vi "Find_Unsigned_Tracks-1.vi"(4 "error IN":errorcluster, 7 "Track ID IN":u16[](array[numeric])) -> (0 "error OUT":errorcluster, 2 "Position Mis ID":i32[](array[numeric]), 3 "Mistake ID":u16[](array[numeric]))   [LabVIEW 2013]
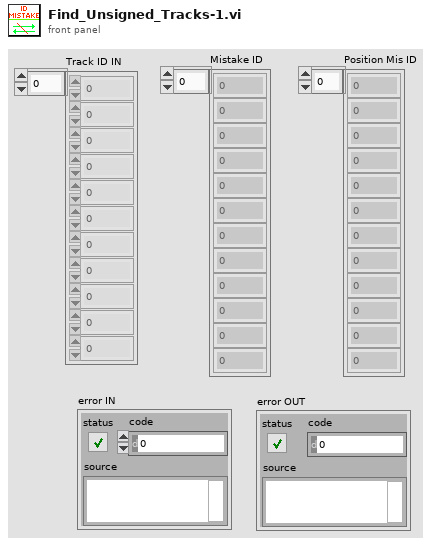
[diagram p1: front panel]
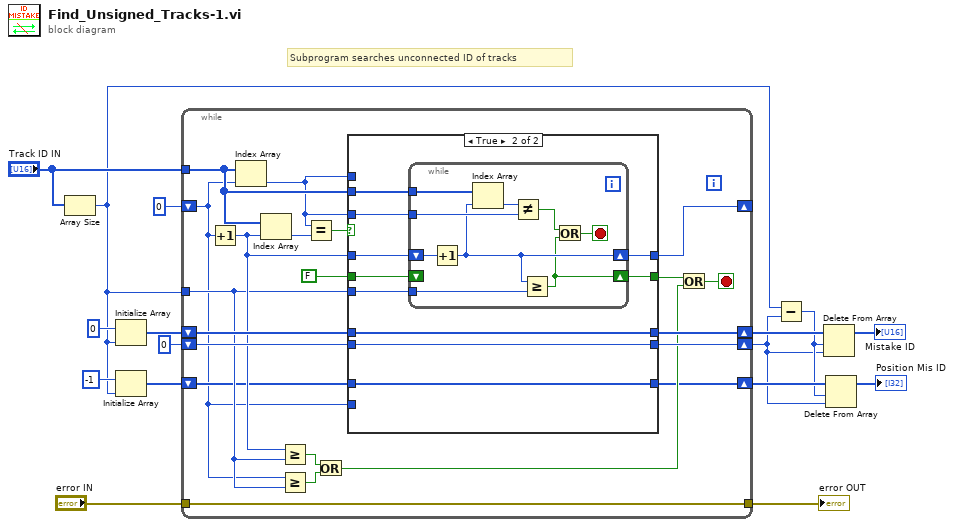
[diagram p0: block diagram]
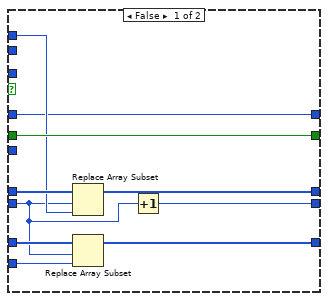
[diagram p2: hidden frame]
diagram:
  # "Subprogram searches unconnected ID of tracks"
  n1 = Array Size(array="Track ID IN") -> (size(s)=w6:i32)
  n2 = Initialize Array(u16 0 ("element"), w6) -> (w14:u16[])
  n3 = Initialize Array(-1 ("element"), w6) -> (w5:i32[])
  n4 = while {
    tunnel: "Track ID IN" -> [w35]
    shift-right: [w29] -> w10
    shift-left: w14 -> [w33]
    shift-right: [w23] -> _
    shift-left: 0 -> [w17]
    tunnel: w6 -> [w27]
    shift-right: [w30] -> w2
    shift-left: 0 -> [w32]
    tunnel: "error IN" -> [w24]
    tunnel: [w24] -> w9
    shift-right: [w18] -> w4
    shift-left: w5 -> [w19]
    stop <- w21 stop-if-true
    n5 = Increment(x=w17) -> (x+1=w28:i32)
    n6 = Index Array(array=w35, index=w17) -> (element=w31:u16)
    n7 = Index Array(array=w35, index=w28) -> (element=w37:u16)
    n8 = Greater Or Equal?(x=w28, y=w27) -> (x >= y?=w26:bool)
    n9 = Greater Or Equal?(x=w17, y=w27) -> (x >= y?=w25:bool)
    n10 = Equal?(x=w31, y=w37) -> (x = y?=w36:bool)
    n11 = Or(x=w26, y=w25) -> (x .or. y?=w20:bool)
    n12 = case shown="True" w36 {
      tunnel: w28 -> [w42 w57]
      tunnel: w35 -> [_ w56]
      tunnel: w31 -> [_ w55]
      tunnel: w27 -> [_ w54]
      tunnel: FALSE -> [w47 w53]
      tunnel: [w47 w50] -> w22
      tunnel: w33 -> [w46 w52]
      tunnel: w32 -> [w38 w51]
      tunnel: w31 -> [w45 _]
      tunnel: [w44 w51] -> w30
      tunnel: [w43 w52] -> w29
      tunnel: [w42 w49] -> w23
      tunnel: w19 -> [w41 w48]
      tunnel: [w40 w48] -> w18
      tunnel: w17 -> [w39 _]
      frame False {
        n13 = Replace Array Subset(array=w46, new element=w45, index=w38) -> (w43:u16[])
        n14 = Replace Array Subset(array=w41, new element=w39, index=w38) -> (w40:i32[])
        n15 = Increment(x=w38) -> (x+1=w44:i32)
      }
      frame True {
        n16 = while {
          shift-right: [w62] -> w49
          shift-left: w57 -> [w66]
          tunnel: w56 -> [w65]
          tunnel: w55 -> [w63]
          tunnel: w54 -> [w61]
          shift-right: [w58] -> w50
          shift-left: w53 -> [_]
          stop <- w59 stop-if-true
          n17 = Increment(x=w66) -> (x+1=w62:i32)
          n18 = Index Array(array=w65, index=w62) -> (element=w64:u16)
          n19 = Not Equal?(x=w64, y=w63) -> (x != y?=w60:bool)
          n20 = Greater Or Equal?(x=w62, y=w61) -> (x >= y?=w58:bool)
          n21 = Or(x=w60, y=w58) -> (x .or. y?=w59:bool)
        }
      }
    }
    n22 = Or(x=w22, y=w20) -> (x .or. y?=w21:bool)
  }
  "error OUT" <- w9
  n23 = Subtract(x=w6, y=w2) -> (x-y=w3:i32)
  n24 = Delete From Array(array=w10, length=w3, index=w2) -> (array with subset deleted=→"Mistake ID":u16[])  [unwired: 1 out]
  n25 = Delete From Array(array=w4, length=w3, index=w2) -> (array with subset deleted=→"Position Mis ID":i32[])  [unwired: 1 out]
